vi "实例1.vi"() -> ()   [LabVIEW 2020]
panel:
  out "Image":T1(plugin-control)
  out "File Data Type":i32(ring)=3 items=["1 bit", "2 bits", "4 bits", "8 bits", "12 bits (unsigned)", "16 bits (unsigned)", "16 bits (signed)", "16 bits (RGB chunky)", "24 bits (RGB chunky)", "24 bits (RGB planar)", "32 bits (unsigned)", "32 bits (signed)", "32 bits (RGB chunky)", "32 bits (float)", "48 bits (Complex 2x24 int)", "64 bits (Complex 2x32 float)", "reserved", "24 bits (HSL)", "48 bits (RGB chunky)", "64 bits (RGB chunky)"]
  out "Image Type":T2 items=["Grayscale (U8)", "Grayscale (I16)", "Grayscale (SGL)", "Complex (CSG)", "RGB (U32)", "HSL (U32)", "RGB (U64)", "Grayscale (U16)"]
  in  "Pattern Label":string="Images (*.tif; *.bmp; *.jpg; *.png; *.apd)"
  out "Cancelled?":bool
  in  "Pattern":string="*.tif;*.bmp;*.jpg;*.jp2;*.png;*.apd"
  in  "Default Name":string
  out "Y Resolution":i32
  out "error out":errorcluster
  out "X Resolution":i32
  out "File Type":string
  out "Calibration":T3={"X Step"=1.0, "Y Step"=1.0, "Unit"=enum."Undefined"} {"Y Step" format="%.2f"; "X Step" format="%.2f"}
  out "Path":path
  out "Paths":path[](array[path])
  in  "Start Path":path
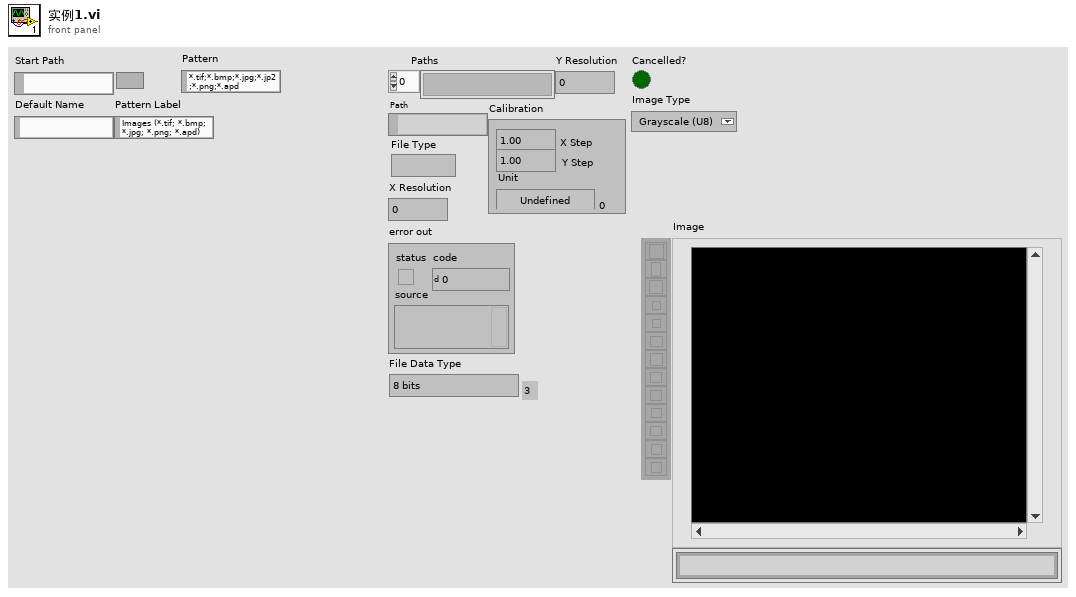
[diagram p1: front panel]
types:
  T1 = typedef "IMAQ Image.ctl" = refnum<image>
  T2 = typedef "Image Type" = u32
  T3 = typedef "Simple Grid Descriptor" = cluster{"X Step":sgl, "Y Step":sgl, "Unit":T4}
  T4 = typedef "Image Unit" = enum32{"Undefined", "Angström", "Micrometer", "Millimeter", "Centimeter", "Meter", "Kilometer", "Microinch", "Inch", "Feet", "Nautical miles", "Standard miles", "Steps"}
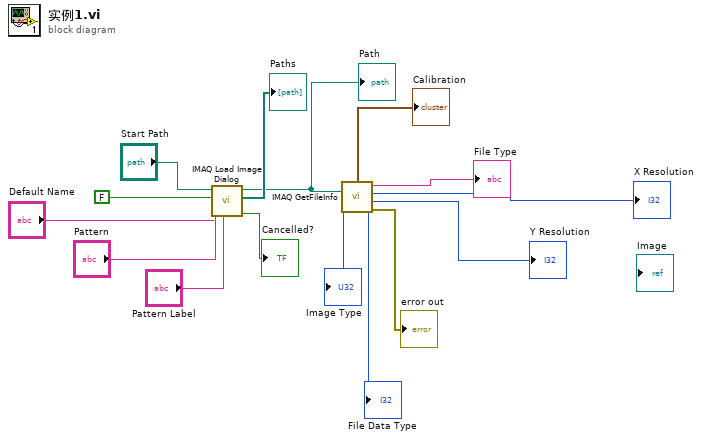
[diagram p0: block diagram]
diagram:
  n1 = call "IMAQ Load Image Dialog"("Pattern Label"="Pattern Label", "Pattern"="Pattern", "Default Name"="Default Name", "Multiple Files? (No)"=FALSE, "Start Path"="Start Path") -> ("Cancelled?"=→"Cancelled?":bool, "Paths"=→"Paths":path[], "Path"=w2:path)  [unwired: 4 in]
  "Path" <- w2
  n2 = call "IMAQ GetFileInfo"("File Path"=w2) -> ("error out"=→"error out":errorcluster, "Y Resolution"=→"Y Resolution":i32, "X Resolution"=→"X Resolution":i32, "File Type"=→"File Type":string, "File Data Type"=→"File Data Type":i32, "Calibration"=→"Calibration":T3, "Image Type"=→"Image Type":T2)  [unwired: 4 in]
